vi "Time_Scales_Tom_Farr.vi"() -> (5 "Plug in titles":string[](array[string]), 7 "Plug in values":string[](array[string]))   [LabVIEW 2010]
uses:
  Globals/Meas_global.vi
  Globals/LDA_meas_global_1.vi
  Globals/Plug_in_data_global.vi
panel:
  out "Time scales":dbl[](array[numeric])
  out "Waveform Graph 2":cluster{dbl, dbl, dbl[]}[](graph)
  out "Waveform Graph":cluster{dbl, dbl, dbl[]}[](graph)
  in  "Data to save":i32[](array[ring])=[1] items=["Pitot (Uref)", "HW (U)", "Save Nothing"]
  # "Run this VI to update the channel names"
  # "You Must have selected the \"Save Data\" option on the \nMeasurement Program for this vi to save time traces"
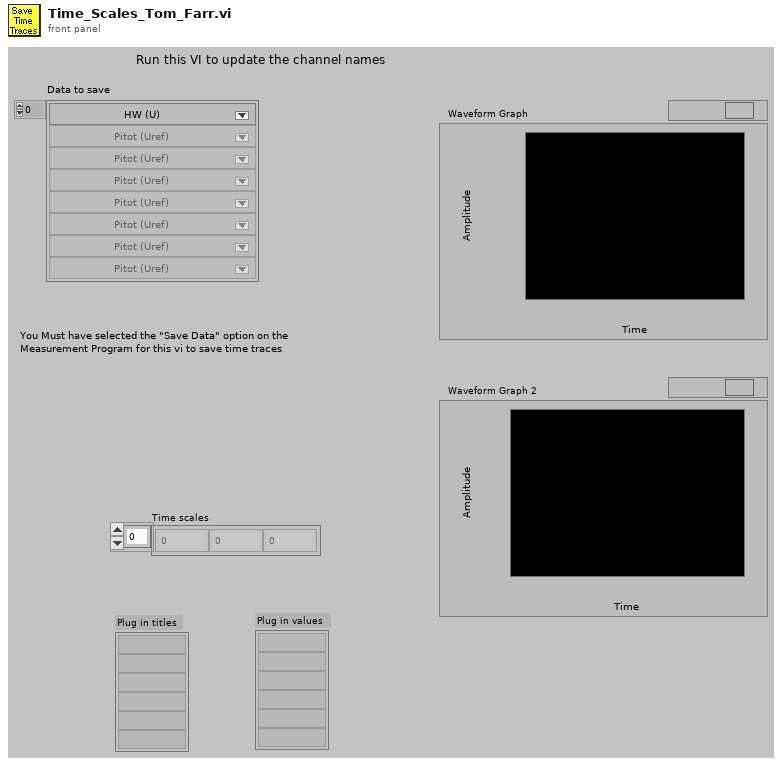
[diagram p1: front panel]
types:
  T1 = typedef "Analysis_info_cluster.ctl" = cluster{"Colour":u32, "Inst type":T2, "Inst name":string, "Symbol":string, "Code name":string, "Extra Info":string, "Inst Array":T3, "Index":i32, "Voltage Index":i32, "Extra Titles":string[], "Extra Values":string[]}
  T2 = typedef "Inst_type.ctl" = enum16{"Propeller anemometer", "Raw voltage", "Pressure Transducer", "Pitot-static tube", "Preston tube", "Hot wire", "Cross wire 1", "Cross wire 2", "Generic Linear", "Generic Polynomial", "Generic BackPoly", "Fast FID", "Thermocouple", "Cold wire", "Pulsed Wire", "LDA Vel", "LDA Tran time", "LDA Arr time"}
  T3 = typedef "Instrument_Array.ctl" = enum16{"PWA", "LDA", "Analogue"}
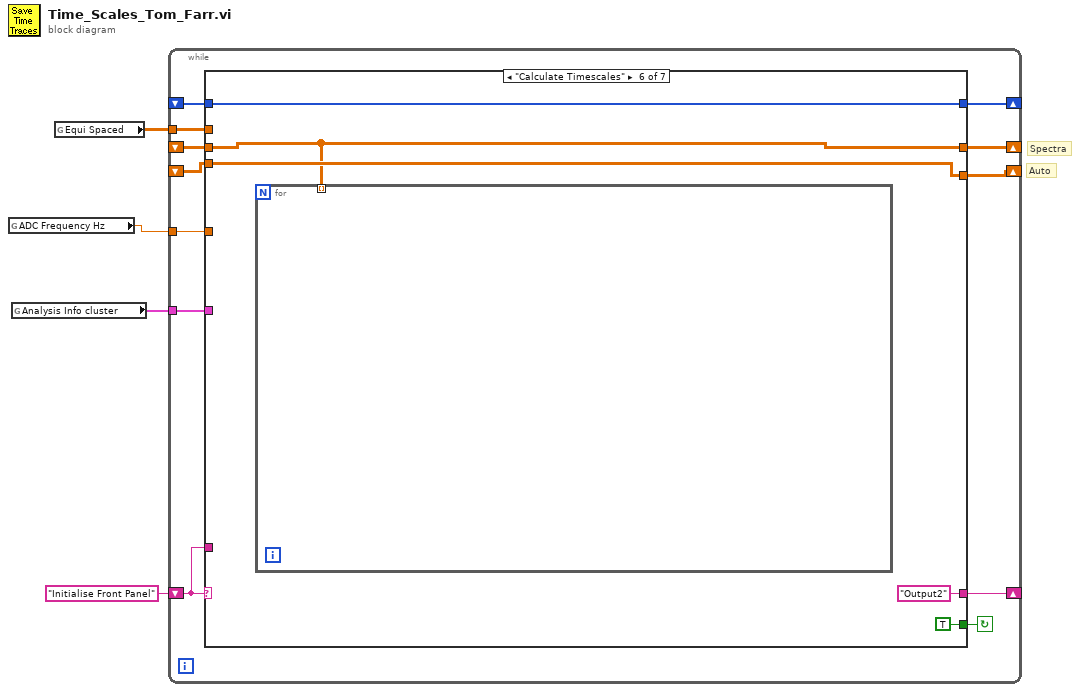
[diagram p0: block diagram]
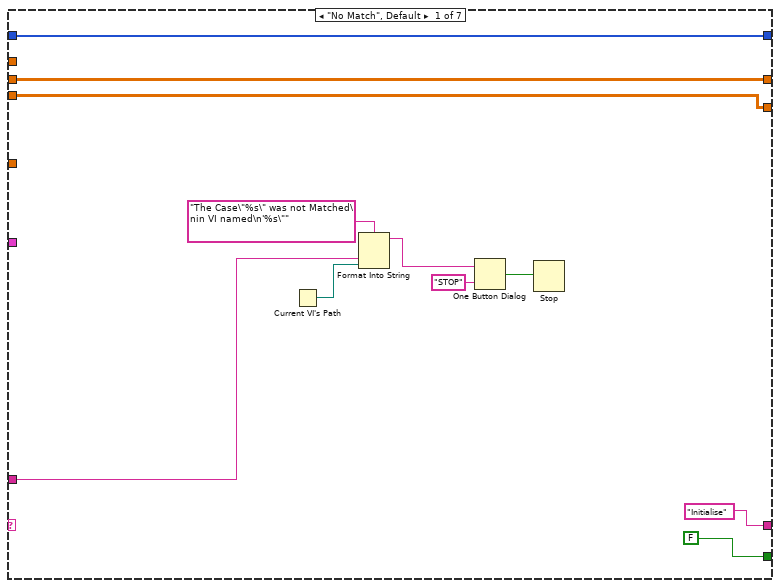
[diagram p2: hidden frame]
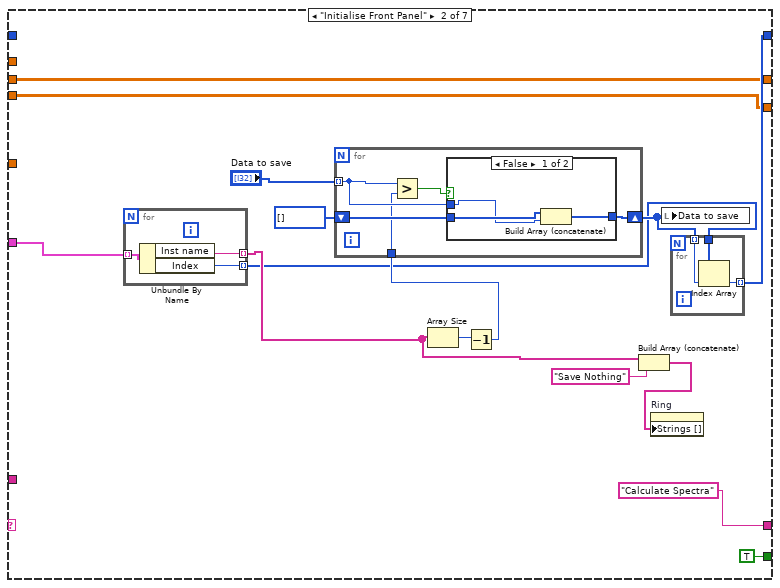
[diagram p3: hidden frame]
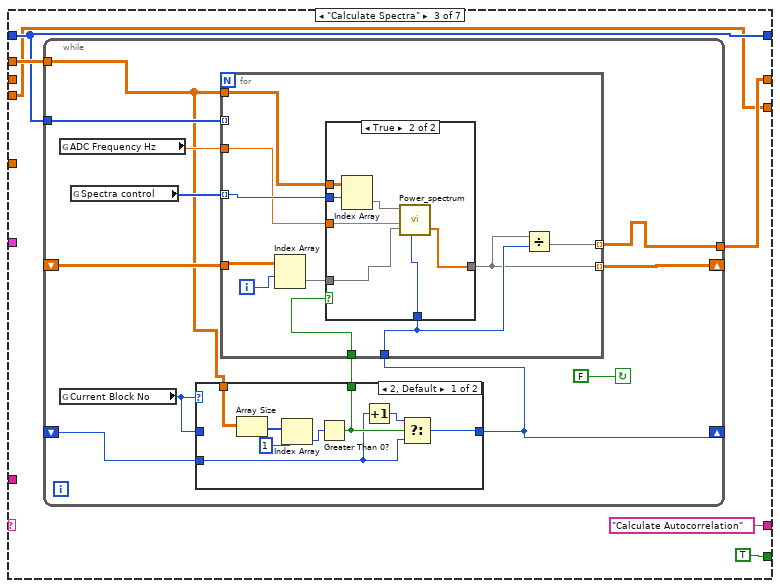
[diagram p5: hidden frame]
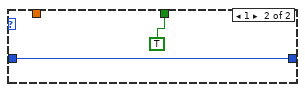
[diagram p6: hidden frame]
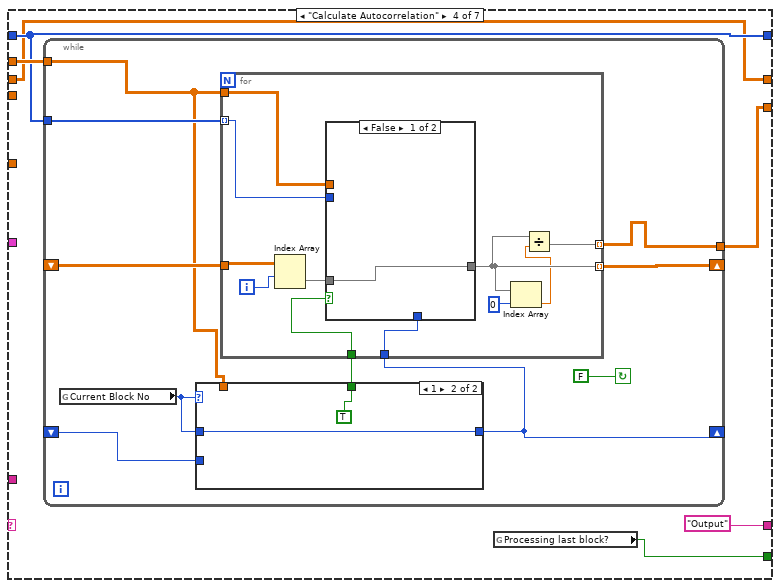
[diagram p8: hidden frame]
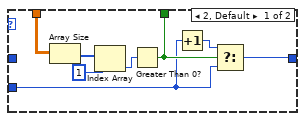
[diagram p9: hidden frame]
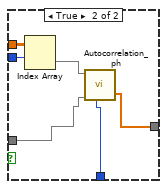
[diagram p10: hidden frame]
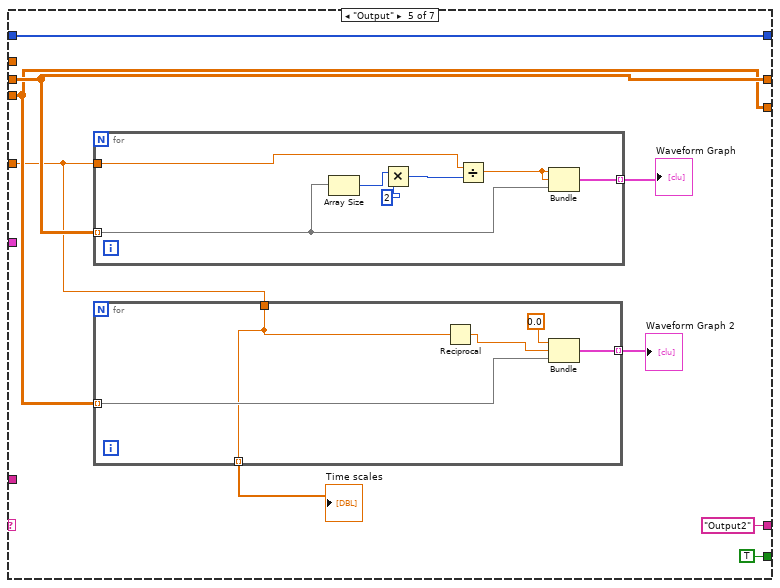
[diagram p11: hidden frame]
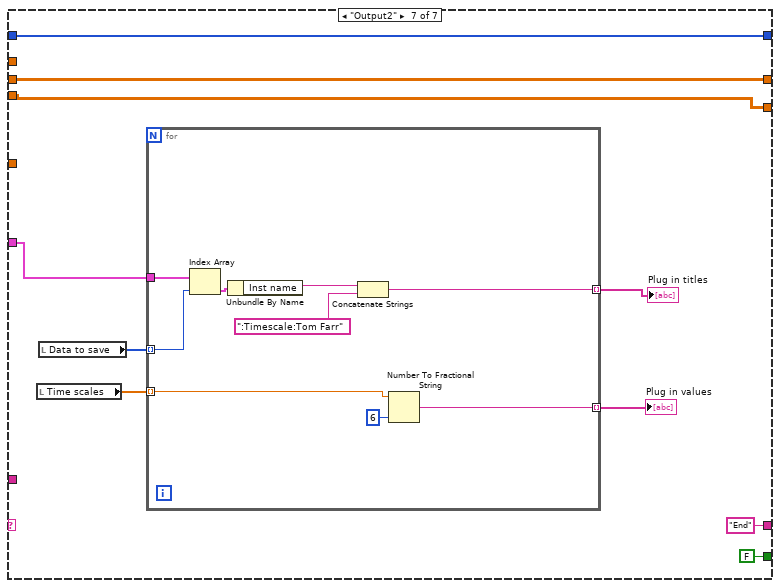
[diagram p12: hidden frame]
diagram:
  # "Spectra"
  # "Auto"
  n1 = global read "LDA_meas_global_1.vi" "ADC Frequency Hz"() -> (w1:dbl)
  n2 = global read "Meas_global.vi" "Analysis Info cluster"() -> (w3:T1[])
  n3 = global read "Plug_in_data_global.vi" "Equi Spaced"() -> (w2:dbl[][])
  n4 = while {
    shift-left: "Initialise Front Panel" -> [w14]
    shift-right: [w15] -> _
    tunnel: w3 -> [w13]
    shift-right: [w12] -> _
    shift-left: _ -> [w9]
    tunnel: w2 -> [w11]
    shift-right: [w10] -> _
    shift-left: _ -> [w8]
    shift-right: [w7] -> _
    shift-left: _ -> [w6]
    tunnel: w1 -> [w5]
    stop <- w16 continue-if-true
    n5 = case shown="\"Calculate Timescales\"" w14 {
      tunnel: [FALSE TRUE TRUE w104 TRUE TRUE FALSE] -> w16
      tunnel: ["Initialise" "Calculate Spectra" ("t") "Calculate Autocorrelation" ("t") "Output" ("t") "Output2" ("t") "Output2" ("t") "End" ("t")] -> w15
      tunnel: w14 -> [w22 _ _ _ _ _ _]
      tunnel: w13 -> [_ w42 _ _ _ _ w179]
      tunnel: [w19 w32 w60 w108 w155 w173 w184] -> w12
      tunnel: w11 -> [_ _ w61 w109 _ _ _]
      tunnel: w9 -> [w19 _ w60 w108 w155 w173 w184]
      tunnel: [w18 w30 w59 w106 w154 w169 w183] -> w10
      tunnel: w8 -> [w18 w30 _ w106 w154 w169 w183]
      tunnel: [w17 w28 w58 w107 w150 w170 w180] -> w7
      tunnel: w6 -> [w17 w28 w58 _ w150 w170 w180]
      tunnel: w5 -> [_ _ _ _ w149 _ _]
      frame "No Match", Default {
        n6 = Current VI's Path() -> (path=w21:path)
        n7 = Format Into String(format string="The Case\"%s\" was not Matched\nin VI named\n'%s\"" ("Format String"), w22, w21) -> (resulting string=w25:string)  [unwired: 2 in, 1 out]
        n8 = One Button Dialog(message=w25, button name ("OK")="STOP") -> (true=w23:bool)
        n9 = Stop(stop? (T)=w23) -> ()
      }
      frame "Initialise Front Panel" {
        n10 = for {
          tunnel: w42 -> [w57] mode=indexing
          tunnel: [w56] -> w36 mode=indexing
          tunnel: [w55] -> w33 mode=indexing
          n11 = Unbundle By Name(w57) -> ("Inst name"=w56:string, "Index"=w55:i32)
        }
        n12 = Array Size(array=w36) -> (size(s)=w38:i32)
        n13 = Decrement(x=w38) -> (x-1=w37:i32)
        n14 = for {
          tunnel: "Data to save" -> [w47] mode=indexing
          shift-right: [w48] -> w34
          shift-left: i32[] [] -> [w49]
          tunnel: w37 -> [w46]
          n15 = Greater?(x=w47, y=w46) -> (0:w50:bool)
          n16 = case shown="False" w50 {
            tunnel: w49 -> [w53 w54]
            tunnel: [w52 w54] -> w48
            tunnel: w47 -> [w51 _]
            frame False {
              n17 = Build Array (concatenate)(w53, w51) -> (w52:i32[])
            }
            frame True {
            }
          }
        }
        n18 = Build Array (concatenate)(w36, "Save Nothing") -> (w39:string[])
        n19 = property on="Ring" class="Ring (strict)"("Strings []"=w39) -> ()  [unwired: 2 in, 2 out]
        n20 = local write "Data to save"(w34) -> ()
        n21 = for {
          tunnel: w34 -> [w45] mode=indexing
          tunnel: w33 -> [w44]
          tunnel: [w43] -> w32 mode=indexing
          n22 = Index Array(array=w44, index=w45) -> (element=w43:i32)
        }
      }
      frame "Calculate Spectra" {
        n23 = while {
          shift-left: _ -> [w73]
          shift-right: [w75] -> _
          shift-right: [w69] -> _
          shift-left: _ -> [w64]
          tunnel: w61 -> [w66]
          tunnel: w60 -> [w67]
          tunnel: [w65] -> w59
          stop <- FALSE continue-if-true
          n24 = global read "LDA_meas_global_1.vi" "ADC Frequency Hz"() -> (w72:dbl)
          n25 = global read "Meas_global.vi" "Current Block No"() -> (w70:i32)
          n26 = global read "Meas_global.vi" "Spectra control"() -> (w74:i32[])
          n27 = case shown="2, Default" w70 {
            tunnel: [w76 w85] -> w69
            tunnel: w70 -> [_ w85]
            tunnel: w66 -> [w83 _]
            tunnel: [w79 TRUE] -> w68
            tunnel: w64 -> [w77 _]
            frame 2, Default {
              n28 = Array Size(array=w83) -> (size(s)=w82:i32[])
              n29 = Index Array(array=w82, index=1) -> (element=w80:i32)
              n30 = Greater Than 0?(x=w80) -> (x > 0?=w79:bool)
              n31 = Increment(x=w77) -> (x+1=w78:i32)
              n32 = Select(t=w78, s=w79, f=w77) -> (s? t:f=w76:i32)
            }
            frame 1 {
            }
          }
          n33 = for {
            tunnel: w74 -> [w94] mode=indexing
            tunnel: w72 -> [w87]
            tunnel: [w89] -> w65 mode=indexing
            tunnel: w69 -> [w95]
            tunnel: [w88] -> w75 mode=indexing
            tunnel: w73 -> [w91]
            tunnel: w68 -> [w93]
            tunnel: w66 -> [w86]
            tunnel: w67 -> [_] mode=indexing
            i -> [w92]
            n34 = Index Array(array=w91, index (row)=w92) -> (element=w90:dbl[])  [unwired: 1 in]
            n35 = case shown="True" w93 {
              tunnel: w87 -> [_ w103]
              tunnel: w95 -> [_ w102]
              tunnel: [w96 w101] -> w88
              tunnel: w86 -> [_ w100]
              tunnel: w94 -> [_ w99]
              tunnel: w90 -> [w96 w98]
              frame False {
              }
              frame True {
                n36 = Index Array(array=w100, index (row)=w99) -> (element=w97:dbl[])  [unwired: 1 in]
                n37 = call "Power_spectrum.vi"("U"=w97, "Sampling frequency"=w103, "Spectrum input array"=w98, "Block No"=w102) -> ("Spectrum output array"=w101:dbl[])  [unwired: 1 in, 1 out]
              }
            }
            n38 = Divide(x=w88, y=w95) -> (x/y=w89:dbl[])
          }
        }
      }
      frame "Calculate Autocorrelation" {
        n39 = while {
          shift-left: _ -> [w118]
          shift-right: [w119] -> _
          shift-right: [w115] -> _
          shift-left: _ -> [w113]
          tunnel: w109 -> [w111]
          tunnel: w108 -> [w112]
          tunnel: [w110] -> w107
          stop <- FALSE continue-if-true
          n40 = global read "Meas_global.vi" "Current Block No"() -> (w116:i32)
          n41 = case shown="1" w116 {
            tunnel: [w120 w129] -> w115
            tunnel: w116 -> [_ w129]
            tunnel: w111 -> [w127 _]
            tunnel: [w123 TRUE] -> w114
            tunnel: w113 -> [w121 _]
            frame 2, Default {
              n42 = Array Size(array=w127) -> (size(s)=w126:i32[])
              n43 = Index Array(array=w126, index=1) -> (element=w124:i32)
              n44 = Greater Than 0?(x=w124) -> (x > 0?=w123:bool)
              n45 = Increment(x=w121) -> (x+1=w122:i32)
              n46 = Select(t=w122, s=w123, f=w121) -> (s? t:f=w120:i32)
            }
            frame 1 {
            }
          }
          n47 = for {
            tunnel: [w136] -> w110 mode=indexing
            tunnel: w115 -> [w132]
            tunnel: [w133] -> w119 mode=indexing
            tunnel: w118 -> [w138]
            tunnel: w114 -> [w140]
            tunnel: w111 -> [w135]
            tunnel: w112 -> [w130] mode=indexing
            i -> [w139]
            n48 = Index Array(array=w138, index (row)=w139) -> (element=w137:dbl[])  [unwired: 1 in]
            n49 = case shown="False" w140 {
              tunnel: w132 -> [_ w142]
              tunnel: [w141 w143] -> w133
              tunnel: w135 -> [_ w147]
              tunnel: w130 -> [_ w146]
              tunnel: w137 -> [w141 w144]
              frame False {
              }
              frame True {
                n50 = Index Array(array=w147, index (row)=w146) -> (element=w145:dbl[])  [unwired: 1 in]
                n51 = call "Autocorrelation_ph.vi"("X"=w145, "Autocorrelation of X"=w144, "Block No"=w142) -> ("Autocorrelation of X"=w143:dbl[])  [unwired: 2 in, 1 out]
              }
            }
            n52 = Index Array(array=w133, index=0 ("Index")) -> (element=w131:dbl)
            n53 = Divide(x=w133, y=w131) -> (x/y=w136:dbl[])
          }
        }
        n54 = global read "Meas_global.vi" "Processing last block?"() -> (w104:bool)
      }
      frame "Output" {
        n55 = for {
          tunnel: w154 -> [w165] mode=indexing
          tunnel: [w166] -> w156 mode=indexing
          tunnel: w149 -> [w162]
          n56 = Array Size(array=w165) -> (size(s)=w164:i32)
          n57 = Multiply(x=w164, y=2) -> (x*y=w168:i32)
          n58 = Divide(x=w162, y=w168) -> (x/y=w167:dbl)
          n59 = Bundle(w167, w167, w165) -> (w166:cluster{dbl, dbl, dbl[]})  [unwired: 1 out]
        }
        "Waveform Graph" <- w156
        n60 = for {
          tunnel: w150 -> [w160] mode=indexing
          tunnel: [w161] -> w151 mode=indexing
          tunnel: w149 -> [w157]
          tunnel: [w157] -> w148 mode=indexing
          n61 = Reciprocal(x=w157) -> (1/x=w158:dbl)
          n62 = Bundle("x/y"=0.0, w158, w160) -> (w161:cluster{"x/y":dbl, dbl, dbl[]})  [unwired: 1 out]
        }
        "Waveform Graph 2" <- w151
        "Time scales" <- w148
      }
      frame "Calculate Timescales" {
        n63 = for {
          tunnel: w169 -> [w174] mode=indexing
        }
      }
      frame "Output2" {
        n64 = local read "Time scales"() -> (w176:dbl[])
        n65 = local read "Data to save"() -> (w178:i32[])
        n66 = for {
          tunnel: w179 -> [w193]
          tunnel: w178 -> [w192] mode=indexing
          tunnel: [w188] -> w177 mode=indexing
          tunnel: w176 -> [w186] mode=indexing
          tunnel: [w185] -> w175 mode=indexing
          n67 = Index Array(array=w193, index=w192) -> (element=w191:T1)
          n68 = Unbundle By Name(w191) -> ("Inst name"=w190:string)
          n69 = Concatenate Strings(w190, ":Timescale:Tom Farr" ("string")) -> (w188:string)
          n70 = Number To Fractional String(number=w186, precision (6)=i16 6) -> (F-format string=w185:string)  [unwired: 2 in]
        }
        "Plug in titles" <- w177
        "Plug in values" <- w175
      }
    }
  }
